vi "Read configuration.vi"(8 "error in (no error)":errorcluster, 11 "Device Channel in":refnum<class "Thermo Channel.lvclass">) -> (0 "error out":errorcluster, 2 "configuration":refnum<class "CEF_serializable configuration.lvclass">, 3 "Device Channel out":refnum<class "Thermo Channel.lvclass">)   [LabVIEW 2025, in "Thermo.lvlib" / "Thermo Channel.lvclass"]
uses:
  Thermo Channel.lvclass
  Users/Public/Documents/Sandia National Labs/TSS Plugin/CEF.lvlibp/serializable configuration/CEF_serializable configuration.lvclass
  Thermo Channel.lvclass/Thermo Channel.ctl
  Thermo Channel configuration/Thermo Channel configuration.lvclass
  C:/Users/Public/Documents/Sandia National Labs/TSS Plugin/CEF.lvlibp/serializable configuration/CEF_serializable configuration.lvclass
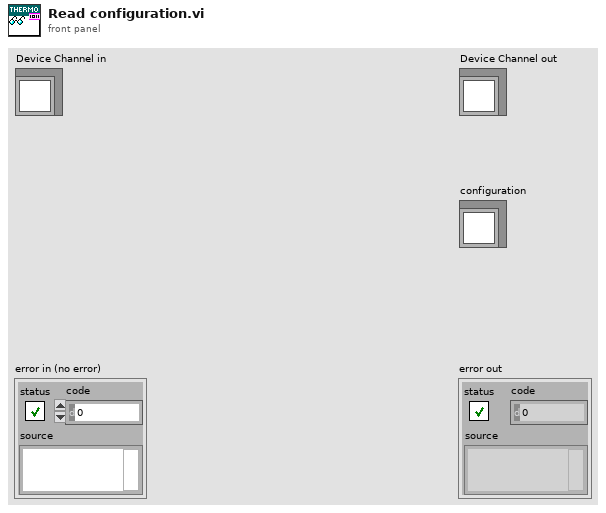
[diagram p1: front panel]
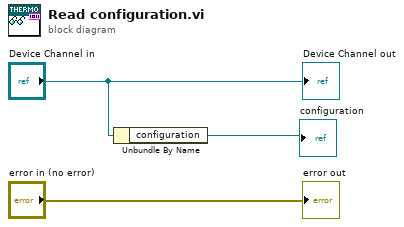
[diagram p0: block diagram]
diagram:
  n1 = Unbundle By Name("Device Channel in") -> ("configuration"=→"configuration":refnum<class "Thermo Channel configuration.lvclass">)
  "error out" <- "error in (no error)"
  "Device Channel out" <- "Device Channel in"
